vi "Configure Analyzer External Attenuation.vi"(7 "External Attenuation (0.0)":dbl format="%.3f", 8 "error in (no error)":errorcluster, 10 "Instance (1)":i32=1 format="%.0g", 11 "VISA resource name":refnum<visa-resource-name>) -> (0 "error out":errorcluster, 3 "VISA resource name out":refnum<visa-resource-name>)   [LabVIEW 2020, in "Rohde&Schwarz CMXP GPRF.lvlib"]
doc: "This VI configures external attenuation value.\n\nAttribute:\nRSCMXPGPRF_ATTR_INPUT_EXTERNAL_ATTENUTATION\n\nRemote-control command:\nCONFigure:GPRF:MEAS<i>:RFSettings:EATTenuation"
uses:
  <instrlib>/Rohde&Schwarz CMXP GPRF/Rohde&Schwarz CMXP GPRF.lvlib
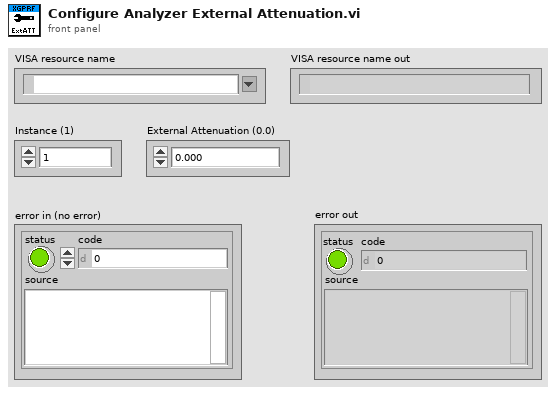
[diagram p1: front panel]
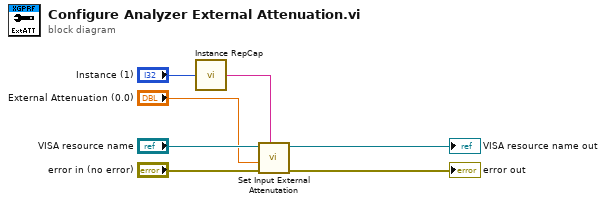
[diagram p0: block diagram]
diagram:
  n1 = call <instrlib>:"Instance RepCap.vi"("Instance in"="Instance (1)") -> ("Instance out"=w4:string)
  n2 = call "Set Input External Attenutation"("Repeated Capabilities"=w4, "error in (no error)"="error in (no error)", "Input External Attenutation (0.0)"="External Attenuation (0.0)", "instrument handle"="VISA resource name") -> ("error out"=→"error out":errorcluster, "instrument handle out"=→"VISA resource name out":refnum<visa-resource-name>)  [unwired: 6 in]
